vi "Load Offsets.vi"(8 "error in (no error)":errorcluster) -> (0 "error out":errorcluster)   [LabVIEW 2009]
uses:
  Apps/App Parameters Actions.ctl
  Logging/LogFileType.ctl
  Data Access Objects/Metadata/Persistant DAO Actions.ctl
  Data Access Objects/Metadata/LBCB Number.ctl
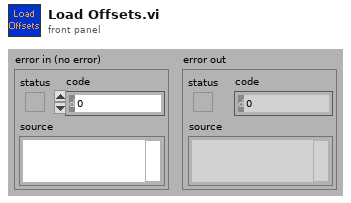
[diagram p1: front panel]
types:
  T1 = typedef "LogFileType.ctl" = enum16{"Continuous", "Step", "Volts", "Offsets", "Mixed Mode State", "DLL  Errors", "End List"}
  T2 = typedef "App Parameters Actions.ctl" = enum16{"Init", "Get", "Set"}
  T3 = typedef "App Parameters.ctl" = cluster{"Monitor Loop":T4, "Ramp Time":T4, "Log Loop":T4, "TCP to DAQ":T4, "Logging Directory":path, "Log File Size (MBytes)":i64, "Volt Logging Loop":T4}
  T4 = typedef "Timing Parameters.ctl" = cluster{"Interval":dbl, "Rate ":dbl}
  T5 = typedef "Persistant DAO Actions.ctl" = enum16{"Init", "Get", "Set", "Load", "Save"}
  T6 = typedef "LBCB Number.ctl" = enum16{"LBCB1", "LBCB2"}
  T7 = typedef "Number Of LBCBs.ctl" = enum16{"1", "2"}
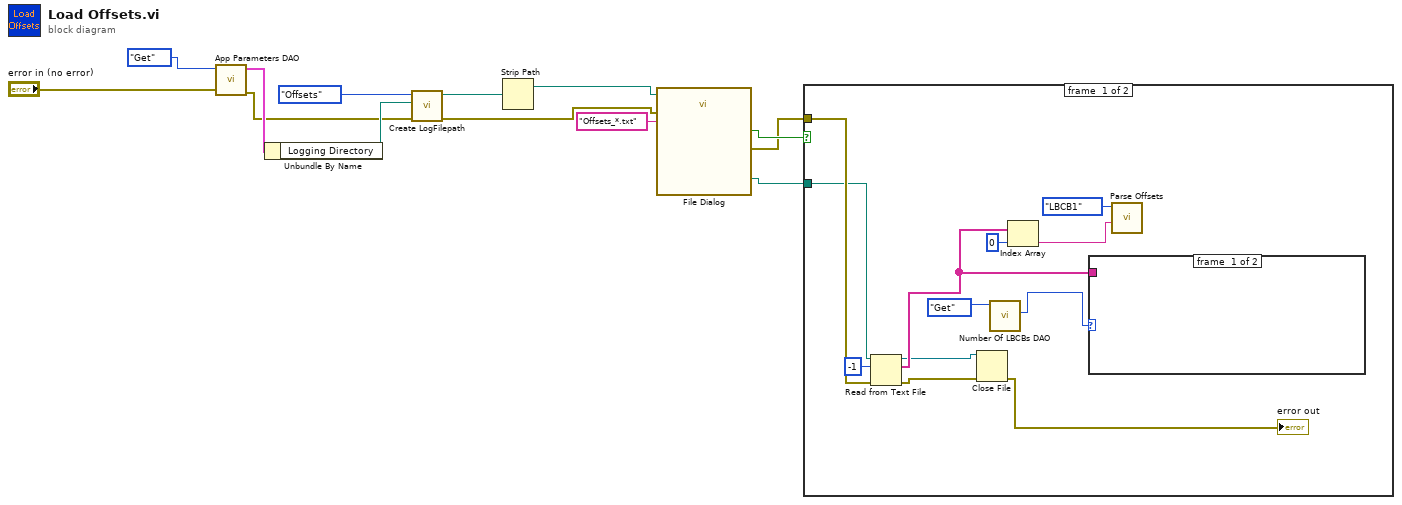
[diagram p0: block diagram]
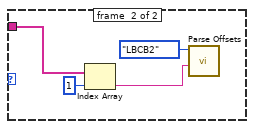
[diagram p2: hidden frame]
diagram:
  n1 = call "App Parameters DAO.vi"("error in (no error)"="error in (no error)", "Actions"=App_Parameters_Actions."Get" ("App Parameter Actions")) -> ("error out"=w10:errorcluster, "Application Timing and Logging Out"=w13:T3)  [unwired: 2 in, 6 out]
  n2 = Unbundle By Name(w13) -> ("Logging Directory"=w12:path)
  n3 = call "Create LogFilepath.vi"("error in (no error)"=w10, "Log Directory"=w12, "LogFile Type"=LogFileType."Offsets") -> ("error out"=w2:errorcluster, "Logfile Path"=w7:path)  [unwired: 7 out]
  n4 = Strip Path(path=w7) -> (stripped path=w5:path)  [unwired: 1 out]
  n5 = call "File Dialog"("start path"=w5, "error in"=w2, "pattern (all files)"="Offsets_*.txt") -> ("selected path"=w6:path, "cancelled"=w3:bool, "error out"=w1:errorcluster)  [unwired: 9 in, 1 out]
  n6 = case shown="False" w3 {
    tunnel: w1 -> [w25 _]
    tunnel: w6 -> [w24 _]
    frame #0 {
      n7 = Read from Text File(file (use dialog)=w24, count=-1, error in=w25) -> (refnum out=w18:refnum<file>, text=w19:string[], error out=w17:errorcluster)  [unwired: 1 in, 1 out]
      n8 = Close File(refnum=w18, error in=w17) -> (error out=→"error out":errorcluster)  [unwired: 1 out]
      n9 = call "Number Of LBCBs DAO.vi"("Actions"=Persistant_DAO_Actions."Get") -> ("Number of\nLBCBs Out"=w14:T7)  [unwired: 8 in, 2 out]
      n10 = Index Array(array=w19, index=0) -> (element=w21:string)
      n11 = case shown="\"2\"" w14 {
        tunnel: w19 -> [_ w26]
        frame #0 {
        }
        frame #1 {
          n12 = Index Array(array=w26, index=1) -> (element=w28:string)
          n13 = call "Parse Offsets.vi"("Line"=w28, "LBCB Selected"=LBCB_Number."LBCB2") -> ()  [unwired: 10 in]
        }
      }
      n14 = call "Parse Offsets.vi"("Line"=w21, "LBCB Selected"=LBCB_Number."LBCB1") -> ()  [unwired: 10 in]
    }
    frame #1 {
    }
  }
